vi "Test setup for MCCW.vi"   [LabVIEW 2020]
uses:
  VSG-SMBV.lvclass
  C:/Sandbox/RF Bench/Source Code/WiSpry Test Framework/Instruments/Instrument.lvclass
  Instrument.lvclass/Instrument.ctl
  Instrument.lvclass
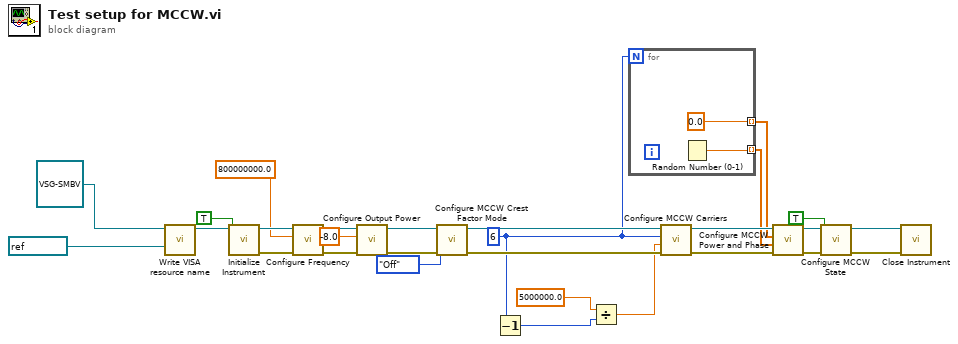
[diagram p0: block diagram]
diagram:
  w8 = 6 ("MCCW Carriers")
  n1 = call "Write VISA resource name.vi"("VISA resource name"=refnum<visa-resource-name> "SMBV", "Instrument in"=refnum<class "VSG-SMBV.lvclass"> refnum ("VSG-SMBV.lvclass")) -> ("Instrument out"=w26:refnum<class "VSG-SMBV.lvclass">)  [unwired: 9 in]
  n2 = call-dynamic "Initialize Instrument.vi"("Reset"=TRUE, "SigGen-SMBV in"=w26) -> ("error out"=w24:errorcluster, "SigGen-SMBV out"=w23:refnum<class "VSG-SMBV.lvclass">)  [unwired: 8 in]
  n3 = call-dynamic "Configure Frequency.vi"("error in (no error)"=w24, "Frequency [Hz]"=800000000.0, "SigGen-SMBV in"=w23) -> ("error out"=w21:errorcluster, "SigGen-SMBV out"=w22:refnum<class "VSG-SMBV.lvclass">)  [unwired: 7 in]
  n4 = call-dynamic "Configure Output Power.vi"("error in (no error)"=w21, "Output Power [dBm]"=-8.0, "SigGen-SMBV in"=w22) -> ("error out"=w18:errorcluster, "SigGen-SMBVout"=w17:refnum<class "VSG-SMBV.lvclass">)  [unwired: 7 in]
  n5 = call-dynamic "Configure MCCW Crest Factor Mode.vi"("error in (no error)"=w18, "Crest factor mode"=enum16{"Off", "Chirp", "Slow"}."Off", "VSG-SMBV in"=w17) -> ("error out"=w15:errorcluster, "VSG-SMBV out"=w14:refnum<class "VSG-SMBV.lvclass">)  [unwired: 7 in]
  n6 = Decrement(x=w8) -> (x-1=w12:i32)
  n7 = Divide(x=5000000.0, y=w12) -> (x/y=w11:dbl)
  n8 = for {
    N: w8 -> [_]
    tunnel: [0.0] -> w7 mode=indexing
    tunnel: [w29] -> w6 mode=indexing
    n9 = Random Number (0-1)() -> (number: 0 to 1=w29:dbl)
  }
  n10 = call-dynamic "Configure MCCW Carriers.vi"("error in (no error)"=w15, "MCCW Carrier spacing [Hz]"=w11, "MCCW Carriers"=w8, "VSG-SMBV in"=w14) -> ("error out"=w9:errorcluster, "VSG-SMBV out"=w10:refnum<class "VSG-SMBV.lvclass">)  [unwired: 6 in]
  n11 = call-dynamic "Configure MCCW Power and Phase.vi"("error in (no error)"=w9, "Phase"=w6, "Power"=w7, "VSG-SMBV in"=w10) -> ("error out"=w5:errorcluster, "VSG-SMBV out"=w4:refnum<class "VSG-SMBV.lvclass">)  [unwired: 6 in]
  n12 = call-dynamic "Configure MCCW State.vi"("error in (no error)"=w5, "State"=TRUE, "VSG-SMBV in"=w4) -> ("error out"=w2:errorcluster, "VSG-SMBV out"=w1:refnum<class "VSG-SMBV.lvclass">)  [unwired: 7 in]
  n13 = call-dynamic "Close Instrument.vi"("error in (no error)"=w2, "Instrument in"=w1) -> ()  [unwired: 8 in, 2 out]
